vi "SwerveDriveMain.vi"(0 "SwerveDriveDevRef":T1={"DevStatus"={"status"=FALSE, "code"=0, "source"=""}, "TurnMotors[]"=[], "Square Inputs"=FALSE, "Max Output"=1.0, "DriveMotors[]"=[], "WheelOffset[]"=[], "SwerveSensors[]"=[], "RobotSize"={"Width"=[], "Length"=[], "Center"=[]}}, 1 "Gyro Angle":dbl, 5 "X":dbl, 7 "Y":dbl, 9 "Z":dbl, 11 "error in (no error)":errorcluster, 12 "Auto":bool, 13 "Robot/ Field Centric":bool) -> (4 "SwerveDriveDevRef":T1={"DevStatus"={"status"=FALSE, "code"=0, "source"=""}, "TurnMotors[]"=[], "Square Inputs"=FALSE, "Max Output"=1.0, "DriveMotors[]"=[], "WheelOffset[]"=[], "SwerveSensors[]"=[], "RobotSize"={"Width"=[], "Length"=[], "Center"=[]}}, 15 "error out":errorcluster)   [LabVIEW 2019, in "Swerve Drive.lvlib"]
uses:
  Swerve Drive.lvlib
  SwerveDriveDevRef.ctl
  <vilib>/Rock Robotics/WPI/MotorControl/WPI_MotorControlDeviceRef.ctl
  <vilib>/Rock Robotics/WPI/MotorControl/WPI_MotorControlType.ctl
  <vilib>/Rock Robotics/SystemInterfaces/DIO/FPGA_DIOPWMChannel.ctl
  <vilib>/Rock Robotics/WPI/PWM/WPI_PWMDeadband.ctl
  <vilib>/Rock Robotics/SystemInterfaces/DIO/FPGA_DIOChannel.ctl
  <vilib>/Rock Robotics/SystemInterfaces/AI/FPGA_AIChannel.ctl
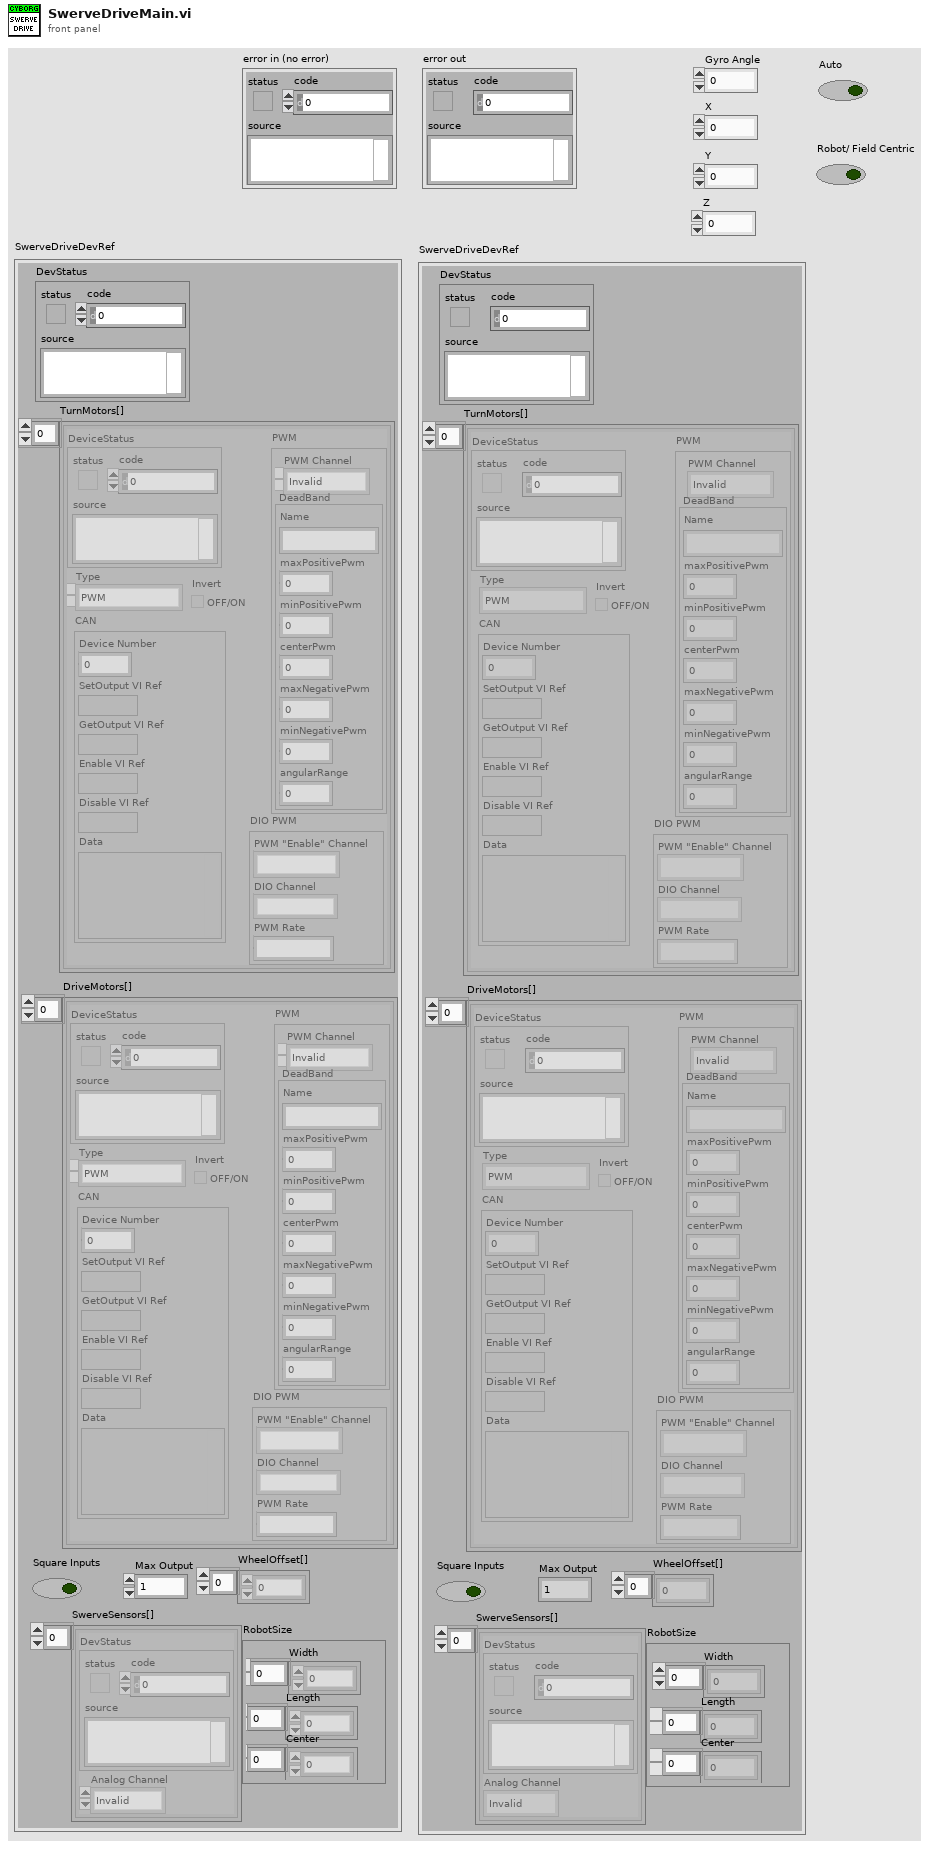
[diagram p1: front panel]
types:
  T1 = typedef "Swerve Drive.lvlib/SwerveDriveDevRef.ctl" = cluster{"DevStatus":errorcluster, "TurnMotors[]":T2[], "Square Inputs":bool, "Max Output":dbl, "DriveMotors[]":T2[], "WheelOffset[]":dbl[], "SwerveSensors[]":cluster{"DevStatus":errorcluster, "Analog Channel":T7}[], "RobotSize":cluster{"Width":dbl[], "Length":dbl[], "Center":dbl[]}}
  T2 = typedef "WPI_MotorControlDeviceRef.ctl" = cluster{"DeviceStatus":errorcluster, "Type":T3, "PWM":cluster{"PWM Channel":T4, "DeadBand":T5}, "CAN":cluster{"Device Number":u8, "SetOutput VI Ref":variant, "GetOutput VI Ref":variant, "Enable VI Ref":variant, "Disable VI Ref":variant, "Data":variant}, "Invert":bool, "DIO PWM":cluster{"PWM \"Enable\" Channel":T4, "DIOChannel":T6, "PWM Rate":dbl}}
  T3 = typedef "WPI_MotorControlType.ctl" = enum16{"PWM", "CAN", "DIO PWM"}
  T4 = typedef "FPGA_DIOPWMChannel.ctl" = enum8{"PWM 0", "PWM 1", "PWM 2", "PWM 3", "PWM 4", "PWM 5", "PWM 6", "PWM 7", "PWM 8", "PWM 9", "PWM MXP 0", "PWM MXP 1", "PWM MXP 2", "PWM MXP 3", "PWM MXP 4", "PWM MXP 5", "PWM MXP 6", "PWM MXP 7", "PWM MXP 8", "PWM MXP 9", "Invalid"}
  T5 = typedef "WPI_PWMDeadband.ctl" = cluster{"Name":string, "maxPositivePwm":i32, "minPositivePwm":i32, "centerPwm":i32, "maxNegativePwm":i32, "minNegativePwm":i32, "angularRange":u16}
  T6 = typedef "FPGA_DIOChannel.ctl" = enum8{"DIO 0", "DIO 1", "DIO 2", "DIO 3", "DIO 4", "DIO 5", "DIO 6", "DIO 7", "DIO 8", "DIO 9", "DIO MXP 0", "DIO MXP 1", "DIO MXP 2", "DIO MXP 3", "DIO MXP 4", "DIO MXP 5", "DIO MXP 6", "DIO MXP 7", "DIO MXP 8", "DIO MXP 9", "DIO MXP 10", "DIO MXP 11", "DIO MXP 12", "DIO MXP 13", "DIO MXP 14", "DIO MXP 15", "SPI Port CS1", "SPI Port CS2", "SPI Port CS3", "SPI Port MISO", "SPI Port MOSI", "Invalid"}
  T7 = typedef "FPGA_AIChannel.ctl" = enum8{"AI 0", "AI 1", "AI 2", "AI 3", "AI MXP 0", "AI MXP 1", "AI MXP 2", "AI MXP 3", "Invalid"}
  T8 = cluster{"DevStatus":errorcluster, "Analog Channel":T7}[]
  T9 = cluster{"Width":dbl[], "Length":dbl[], "Center":dbl[]}
  T10 = cluster{"DevStatus":errorcluster, "Analog Channel":T7}
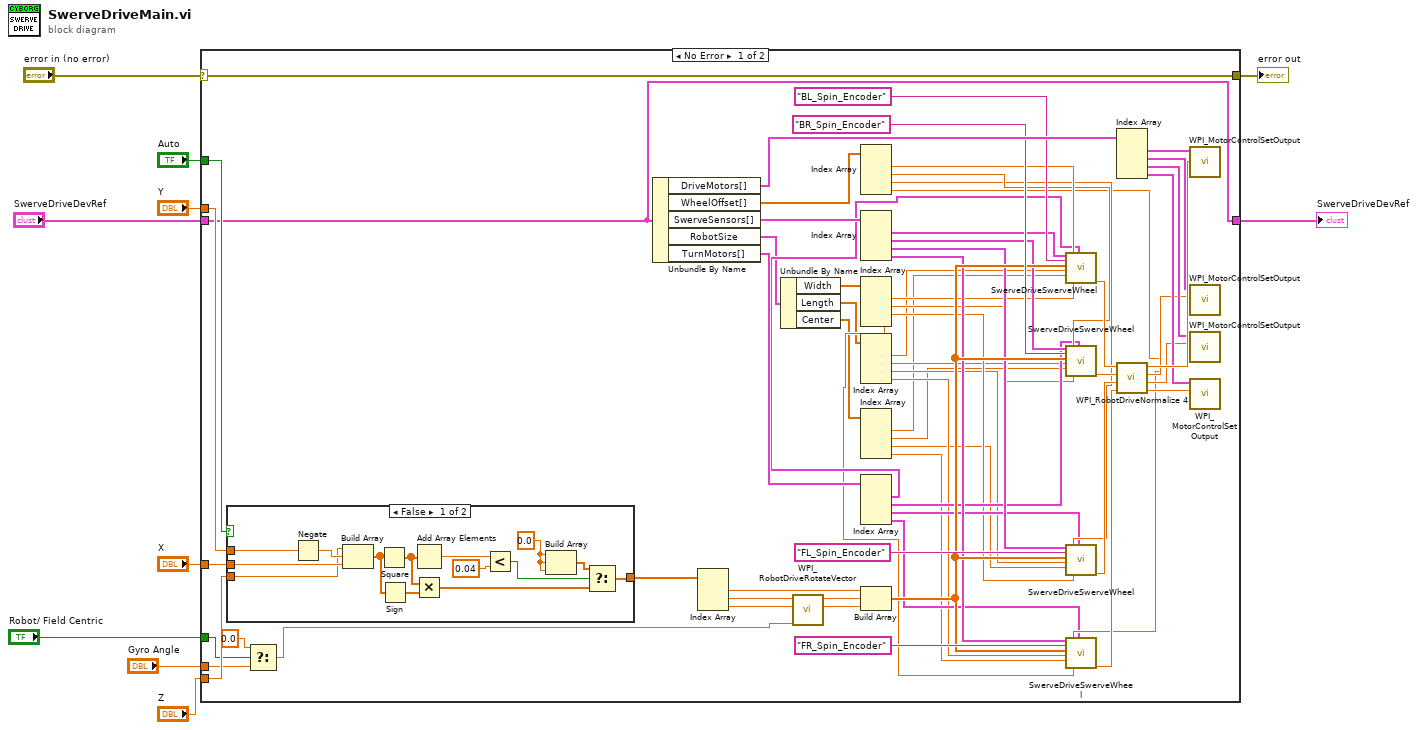
[diagram p0: block diagram]
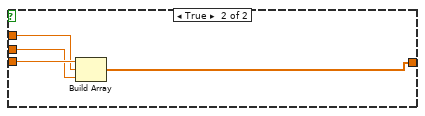
[diagram p2: hidden frame]
diagram:
  n1 = case shown="No Error" "error in (no error)" {
    selector: "error in (no error)" -> [w65 w94]
    tunnel: "SwerveDriveDevRef" -> [w60 w95]
    tunnel: [w60 w95] -> w8
    tunnel: "Z" -> [w72 _]
    tunnel: "Y" -> [w71 _]
    tunnel: "X" -> [w70 _]
    tunnel: "Auto" -> [w69 _]
    tunnel: [w65 w94] -> w3
    tunnel: "Robot/ Field Centric" -> [w64 _]
    tunnel: "Gyro Angle" -> [w62 _]
    frame No Error {
      n2 = case shown="False" w69 {
        tunnel: [w79 w93] -> w73
        tunnel: w72 -> [w76 w92]
        tunnel: w71 -> [w77 w91]
        tunnel: w70 -> [w78 w90]
        frame False {
          w85 = 0.0 ("element")
          n3 = Negate(x=w77) -> (-x=w81:dbl)
          n4 = Build Array(w76, w81, w78) -> (w84:dbl[])
          n5 = Square(x=w84) -> (x^2=w82:dbl[])
          n6 = Sign(1:w84) -> (0:w83:dbl[])
          n7 = Add Array Elements(numeric array=w82) -> (sum=w89:dbl)
          n8 = Multiply(x=w82, y=w83) -> (x*y=w80:dbl[])
          n9 = Less?(x=w89, y=0.04 ("x")) -> (x < y?=w87:bool)
          n10 = Build Array(w85, w85, w85) -> (w86:dbl[])
          n11 = Select(t=w86, s=w87, f=w80) -> (s? t:f=w79:dbl[])
        }
        frame True {
          n12 = Build Array(w92, w91, w90) -> (w93:dbl[])
        }
      }
      n13 = Select(t=0.0, s=w64, f=w62) -> (s? t:f=w61:dbl)
      n14 = Unbundle By Name(w60) -> ("DriveMotors[]"=w59:T2[], "WheelOffset[]"=w41:dbl[], "SwerveSensors[]"=w36:T8, "RobotSize"=w26:T9, "TurnMotors[]"=w31:T2[])
      n15 = Index Array(array=w73) -> (element #1=w68:dbl, element #2=w74:dbl, element #3=w75:dbl)  [unwired: 3 in]
      n16 = Unbundle By Name(w26) -> ("Width"=w25:dbl[], "Length"=w20:dbl[], "Center"=w15:dbl[])
      n17 = call <vilib>:"WPI_RobotDriveRotateVector.vi"("Angle"=w61, "X"=w75, "Y"=w74) -> ("X'"=w66:dbl, "Y'"=w67:dbl)  [unwired: 7 out]
      n18 = Index Array(array=w41) -> (element #1=w40:dbl, element #2=w39:dbl, element #3=w38:dbl, element #4=w37:dbl)  [unwired: 4 in]
      n19 = Index Array(array=w36) -> (element #1=w35:T10, element #2=w34:T10, element #3=w33:T10, element #4=w32:T10)  [unwired: 4 in]
      n20 = Index Array(array=w25) -> (element #1=w24:dbl, element #2=w23:dbl, element #3=w22:dbl, element #4=w21:dbl)  [unwired: 4 in]
      n21 = Index Array(array=w20) -> (element #1=w19:dbl, element #2=w18:dbl, element #3=w17:dbl, element #4=w16:dbl)  [unwired: 4 in]
      n22 = Index Array(array=w15) -> (element #1=w14:dbl, element #2=w13:dbl, element #3=w12:dbl, element #4=w11:dbl)  [unwired: 4 in]
      n23 = Index Array(array=w31) -> (element #1=w30:T2, element #2=w29:T2, element #3=w28:T2, element #4=w27:T2)  [unwired: 4 in]
      n24 = Build Array(w68, w67, w66) -> (w48:dbl[])
      n25 = call "SwerveDriveSwerveWheel.vi"("Wheel_Encoder"=w35, "Wheel_Position"="BL_Spin_Encoder" ("refnum name"), "Inputs"=w48, "Length"=w19, "Center"=w14, "Wheel_Offset"=w40, "Width"=w24, "MotorControlDevRef"=w30) -> ("Speed"=w56:dbl)  [unwired: 11 in]
      n26 = call "SwerveDriveSwerveWheel.vi"("Wheel_Encoder"=w34, "Wheel_Position"="BR_Spin_Encoder" ("refnum name"), "Inputs"=w48, "Length"=w18, "Center"=w13, "Wheel_Offset"=w39, "Width"=w23, "MotorControlDevRef"=w29) -> ("Speed"=w55:dbl)  [unwired: 11 in]
      n27 = call "SwerveDriveSwerveWheel.vi"("Wheel_Encoder"=w33, "Wheel_Position"="FL_Spin_Encoder" ("refnum name"), "Inputs"=w48, "Length"=w17, "Center"=w12, "Wheel_Offset"=w38, "Width"=w22, "MotorControlDevRef"=w28) -> ("Speed"=w54:dbl)  [unwired: 11 in]
      n28 = call "SwerveDriveSwerveWheel.vi"("Wheel_Encoder"=w32, "Wheel_Position"="FR_Spin_Encoder" ("refnum name"), "Inputs"=w48, "Length"=w16, "Center"=w11, "Wheel_Offset"=w37, "Width"=w21, "MotorControlDevRef"=w27) -> ("Speed"=w53:dbl)  [unwired: 11 in]
      n29 = Index Array(array=w59) -> (element #1=w58:T2, element #2=w47:T2, element #3=w46:T2, element #4=w45:T2)  [unwired: 4 in]
      n30 = call <vilib>:"WPI_RobotDriveNormalize 4.vi"("D"=w53, "C"=w54, "B"=w55, "A"=w56) -> ("D'"=w44:dbl, "C'"=w43:dbl, "B'"=w42:dbl, "A'"=w57:dbl)
      n31 = call <vilib>:"WPI_MotorControlSetOutput.vi"("Output"=w57, "MotorControlDevRef"=w58) -> ()  [unwired: 7 in, 3 out]
      n32 = call <vilib>:"WPI_MotorControlSetOutput.vi"("Output"=w42, "MotorControlDevRef"=w47) -> ()  [unwired: 7 in, 3 out]
      n33 = call <vilib>:"WPI_MotorControlSetOutput.vi"("Output"=w43, "MotorControlDevRef"=w46) -> ()  [unwired: 7 in, 3 out]
      n34 = call <vilib>:"WPI_MotorControlSetOutput.vi"("Output"=w44, "MotorControlDevRef"=w45) -> ()  [unwired: 7 in, 3 out]
    }
    frame Error {
    }
  }
  "SwerveDriveDevRef" <- w8
  "error out" <- w3
